vi "svx_Set SampPerChan (DAQmx).vi"(0 "acquisition task in":T1={"AI device settings"={"AI DAQmx TaskID"="", "response"=[]}, "acquisition type"=enum."Finite", "measurement settings"={"AI sampling frequency"=0.0, "AO sampling frequency"=0.0, "AI block size"=0, "AO block Size"=0, "block duration [ms]"=100.0, "number of AI channels"=0, "device propagation delay [samples]"=0.0, "DUT propagation time [s]"=0.0}, "settling settings"={"settle time"=0.0, "settle cycles"=0}, "integration settings"={"integration time"=0.0, "integration cycles"=0}, "AO device settings"={"AO DAQmx taskID"="", "excitation"=[]}, "acquisition accounting"={"initial read size [samples]"=0, "read offset [samples]"=0, "read length [samples]"=0, "blocks to settle [samples]"=0, "min delay until transition [samples]"=0}, "frequency range"={"start frequency"=0.0, "stop frequency"=0.0}, "block type"=enum."Initialize", "source settings"={"signal type"=enum."Sine wave", "frequency"=0.0, "total amplitude"=0.0, "frequencies"=[], "relative amplitudes"=[], "offset"=0.0, "total amplitude list"=[], "ramping rate"=0.0}, "chirp settings"={"amplitude"=1.0, "frequency range"={"start (Hz)"=20.0, "stop (Hz)"=20000.0, "frequency spacing"=enum."Logarithmic"}, "sampling info"={"Fs"=50000.0, "chirp duration [s]"=3.0}, "initial states"={"frequency [Hz]"=20.0, "phase [rad]"=0.0, "elapsed time [s]"=0.0}, "frequency slope"=0.0, "maximum harmonic"=3, "prefix len [samples]"={"integer"=0, "fractional"=0.0}}} {"chirp settings"."frequency slope" format="%.2f"; "chirp settings"."prefix len [samples]"."fractional" format="%.2p"; "chirp settings"."initial states"."elapsed time [s]" format="%.2f"; "chirp settings"."initial states"."phase [rad]" format="%.2f"; "chirp settings"."initial states"."frequency [Hz]" format="%.2f"; "chirp settings"."sampling info"."chirp duration [s]" format="%.2f"; "chirp settings"."sampling info"."Fs" format="%.2p"; "chirp settings"."frequency range"."stop (Hz)" format="%.2f"; "chirp settings"."frequency range"."start (Hz)" format="%.2f"; "chirp settings"."amplitude" format="%.2f"; "source settings"."total amplitude" format="%.2f"; "source settings"."relative amplitudes" format="%.2f"; "source settings"."frequencies" format="%.2f"; "source settings"."total amplitude list" format="%.2f"; "source settings"."ramping rate" format="%.4f"; "source settings"."offset" format="%.2f"; "source settings"."frequency" format="%.2f"; "frequency range"."stop frequency" format="%.2f"; "frequency range"."start frequency" format="%.2f"; "AO device settings"."excitation"."AO channel settings"."terminal config" items=["Default"=-1, "Differential"=10106, "Pseudodifferential"=12529]; "AI device settings"."response"."AI channel settings"."DSA channel settings"."IEPE current [mA]" min=0.0 max=20.0 format="%.1f"; "AI device settings"."response"."AI channel settings"."DSA channel settings"."coupling" items=["AC"=10045, "DC"=10050, "GND"=10066]; "AI device settings"."response"."AI channel settings"."min value [V]" format="%.2f"; "AI device settings"."response"."AI channel settings"."terminal config" items=["Default"=-1, "RSE"=10083, "NRSE"=10078, "Differential"=10106, "Pseudodifferential"=12529]; "AI device settings"."response"."AI channel settings"."max value [V]" format="%.2f"; "integration settings"."integration time" format="%.2p"; "settling settings"."settle time" format="%.2p"; "measurement settings"."DUT propagation time [s]" format="%.2f"; "measurement settings"."AO sampling frequency" format="%.2f"; "measurement settings"."AI sampling frequency" format="%.2f"}, 11 "error in (no error)":errorcluster) -> (4 "acquisition task out":T1={"AI device settings"={"AI DAQmx TaskID"="", "response"=[]}, "acquisition type"=enum."Finite", "measurement settings"={"AI sampling frequency"=0.0, "AO sampling frequency"=0.0, "AI block size"=0, "AO block Size"=0, "block duration [ms]"=100.0, "number of AI channels"=0, "device propagation delay [samples]"=0.0, "DUT propagation time [s]"=0.0}, "settling settings"={"settle time"=0.0, "settle cycles"=0}, "integration settings"={"integration time"=0.0, "integration cycles"=0}, "AO device settings"={"AO DAQmx taskID"="", "excitation"=[]}, "acquisition accounting"={"initial read size [samples]"=0, "read offset [samples]"=0, "read length [samples]"=0, "blocks to settle [samples]"=0, "min delay until transition [samples]"=0}, "frequency range"={"start frequency"=0.0, "stop frequency"=0.0}, "block type"=enum."Initialize", "source settings"={"signal type"=enum."Sine wave", "frequency"=0.0, "total amplitude"=0.0, "frequencies"=[], "relative amplitudes"=[], "offset"=0.0, "total amplitude list"=[], "ramping rate"=0.0}, "chirp settings"={"amplitude"=1.0, "frequency range"={"start (Hz)"=20.0, "stop (Hz)"=20000.0, "frequency spacing"=enum."Logarithmic"}, "sampling info"={"Fs"=50000.0, "chirp duration [s]"=3.0}, "initial states"={"frequency [Hz]"=20.0, "phase [rad]"=0.0, "elapsed time [s]"=0.0}, "frequency slope"=0.0, "maximum harmonic"=3, "prefix len [samples]"={"integer"=0, "fractional"=0.0}}} {"chirp settings"."frequency slope" format="%.2f"; "chirp settings"."prefix len [samples]"."fractional" format="%.2p"; "chirp settings"."initial states"."elapsed time [s]" format="%.2f"; "chirp settings"."initial states"."phase [rad]" format="%.2f"; "chirp settings"."initial states"."frequency [Hz]" format="%.2f"; "chirp settings"."sampling info"."chirp duration [s]" format="%.2f"; "chirp settings"."sampling info"."Fs" format="%.2p"; "chirp settings"."frequency range"."stop (Hz)" format="%.2f"; "chirp settings"."frequency range"."start (Hz)" format="%.2f"; "chirp settings"."amplitude" format="%.2f"; "source settings"."total amplitude" format="%.2f"; "source settings"."relative amplitudes" format="%.2f"; "source settings"."frequencies" format="%.2f"; "source settings"."total amplitude list" format="%.2f"; "source settings"."ramping rate" format="%.4f"; "source settings"."offset" format="%.2f"; "source settings"."frequency" format="%.2f"; "frequency range"."stop frequency" format="%.2f"; "frequency range"."start frequency" format="%.2f"; "AO device settings"."excitation"."AO channel settings"."terminal config" items=["Default"=-1, "Differential"=10106, "Pseudodifferential"=12529]; "AI device settings"."response"."AI channel settings"."DSA channel settings"."IEPE current [mA]" min=0.0 max=20.0 format="%.1f"; "AI device settings"."response"."AI channel settings"."DSA channel settings"."coupling" items=["AC"=10045, "DC"=10050, "GND"=10066]; "AI device settings"."response"."AI channel settings"."min value [V]" format="%.2f"; "AI device settings"."response"."AI channel settings"."terminal config" items=["Default"=-1, "RSE"=10083, "NRSE"=10078, "Differential"=10106, "Pseudodifferential"=12529]; "AI device settings"."response"."AI channel settings"."max value [V]" format="%.2f"; "integration settings"."integration time" format="%.2p"; "settling settings"."settle time" format="%.2p"; "measurement settings"."DUT propagation time [s]" format="%.2f"; "measurement settings"."AO sampling frequency" format="%.2f"; "measurement settings"."AI sampling frequency" format="%.2f"}, 15 "error out":errorcluster)   [LabVIEW 2017]
uses:
  <vilib>/addons/Sound and Vibration/Example Support/Audio/DAQmx/svx_Acquisition Task (DAQmx).ctl
  <vilib>/addons/_NISVFA/_Shared subVIs/Controls/svc_Channel Settings.ctl
  <vilib>/addons/_NISVFA/_Shared subVIs/Controls/svc_DSA Channel Settings.ctl
  <vilib>/addons/_NISVFA/_Generation/subVIs/sv_Chirp Settings.ctl
  <resource>/objmgr/daqmx.rc
  <vilib>/addons/_NISVFA/_Generation/SoundVib_Generation.lvlib
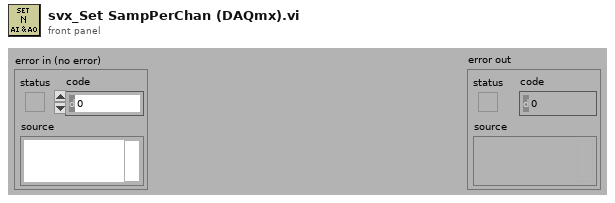
[diagram p1: front panel]
types:
  T1 = typedef "svx_Acquisition Task (DAQmx).ctl" = cluster{"AI device settings":cluster{"AI DAQmx TaskID":refnum<k21>, "response":cluster{"AI physical channel":tag, "AI channel settings":T2}[]}, "acquisition type":enum16{"Finite", "Averaged", "Settled", "Amplitude Sweep", "Stepped Frequency Sweep", "Continuous Frequency Sweep"}, "measurement settings":cluster{"AI sampling frequency":dbl, "AO sampling frequency":dbl, "AI block size":i32, "AO block Size":i32, "block duration [ms]":dbl, "number of AI channels":i32, "device propagation delay [samples]":dbl, "DUT propagation time [s]":dbl}, "settling settings":cluster{"settle time":dbl, "settle cycles":i32}, "integration settings":cluster{"integration time":dbl, "integration cycles":i32}, "AO device settings":cluster{"AO DAQmx taskID":refnum<k21>, "excitation":cluster{"AO physical channel":tag, "AO channel settings":cluster{"maximum value (10 V)":dbl, "minimum value (10 V)":dbl, "terminal config":i32}}[]}, "acquisition accounting":cluster{"initial read size [samples]":i32, "read offset [samples]":i32, "read length [samples]":i32, "blocks to settle [samples]":i32, "min delay until transition [samples]":i32}, "frequency range":cluster{"start frequency":dbl, "stop frequency":dbl}, "block type":enum16{"Initialize", "Settle", "Integrate"}, "source settings":cluster{"signal type":enum16{"Sine wave", "Dual tone (IMD)", "Multitone", "Chirp", "Frequency flat chirp", "Uniform white noise", "Gaussian white noise", "Pink noise", "PRN", "Continuous swept-sine"}, "frequency":dbl, "total amplitude":dbl, "frequencies":dbl[], "relative amplitudes":dbl[], "offset":dbl, "total amplitude list":dbl[], "ramping rate":dbl}, "chirp settings":T4}
  T2 = typedef "svc_Channel Settings.ctl" = cluster{"max value [V]":dbl, "min value [V]":dbl, "terminal config":i32, "DSA channel settings":T3}
  T3 = typedef "svc_DSA Channel Settings.ctl" = cluster{"coupling":i32, "enable IEPE excitation":bool, "IEPE current [mA]":dbl}
  T4 = typedef "SoundVib_Generation.lvlib/sv_Chirp Settings.ctl" = cluster{"amplitude":dbl, "frequency range":cluster{"start (Hz)":dbl, "stop (Hz)":dbl, "frequency spacing":enum16{"Linear", "Logarithmic"}}, "sampling info":cluster{"Fs":dbl, "chirp duration [s]":dbl}, "initial states":cluster{"frequency [Hz]":dbl, "phase [rad]":dbl, "elapsed time [s]":dbl}, "frequency slope":dbl, "maximum harmonic":i32, "prefix len [samples]":cluster{"integer":u32, "fractional":dbl}}
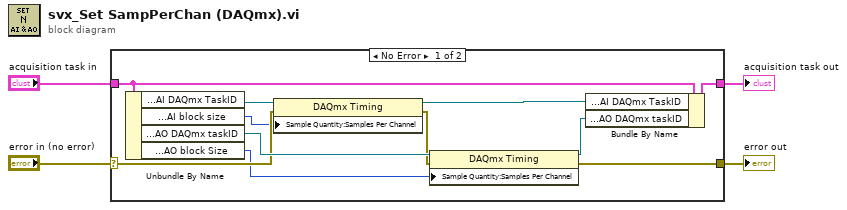
[diagram p0: block diagram]
diagram:
  n1 = case shown="No Error" "error in (no error)" {
    selector: "error in (no error)" -> [w7 w16]
    tunnel: "acquisition task in" -> [w14 w17]
    tunnel: [w9 w17] -> w3
    tunnel: [w8 w16] -> w2
    frame No Error {
      n2 = Unbundle By Name(w14) -> ("AI device settings.AI DAQmx TaskID"=w13:refnum<k21>, "measurement settings.AI block size"=w6:i32, "AO device settings.AO DAQmx taskID"=w12:refnum<k21>, "measurement settings.AO block Size"=w5:i32)
      n3 = property class="DAQmx Timing"(reference=w13, error in=w7, "Sample Quantity:Samples Per Channel"=w6) -> (reference out=w15:refnum<k21>, error out=w10:errorcluster)
      n4 = property class="DAQmx Timing"(reference=w12, error in=w10, "Sample Quantity:Samples Per Channel"=w5) -> (reference out=w11:refnum<k21>, error out=w8:errorcluster)
      n5 = Bundle By Name(cluster=w14, "AI device settings.AI DAQmx TaskID"=w15, "AO device settings.AO DAQmx taskID"=w11) -> (w9:T1)
    }
    frame Error {
    }
  }
  "acquisition task out" <- w3
  "error out" <- w2
